vi "Get Error Source Components.vi"(11 "Error Source String":string) -> (1 "DQMH Error Hint":string, 2 "Call Chain":string[](array[string]), 3 "Error Message":string)   [LabVIEW 2024, in "hse-logger.lvlib" / "Formatter.lvclass"]
doc: "Extract the call chain from extended source strings.\n\n____\nHAMPEL SOFTWARE ENGINEERING v2.2.2 (2025-01-16 15:41)"
uses:
  <vilib>/Hampel Software Engineering/HSE Logger/Formatter/Formatter.lvclass
  <vilib>/Utility/error.llb/Trim Whitespace One-Sided.vi
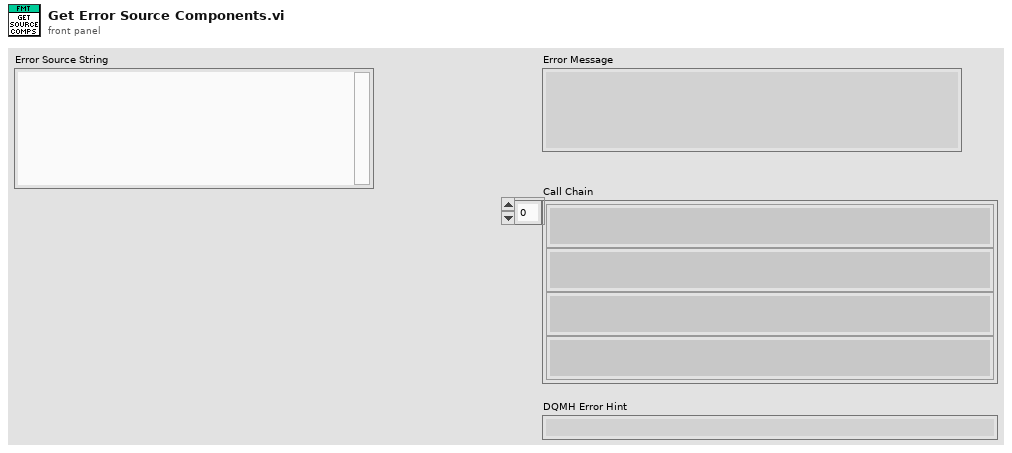
[diagram p1: front panel]
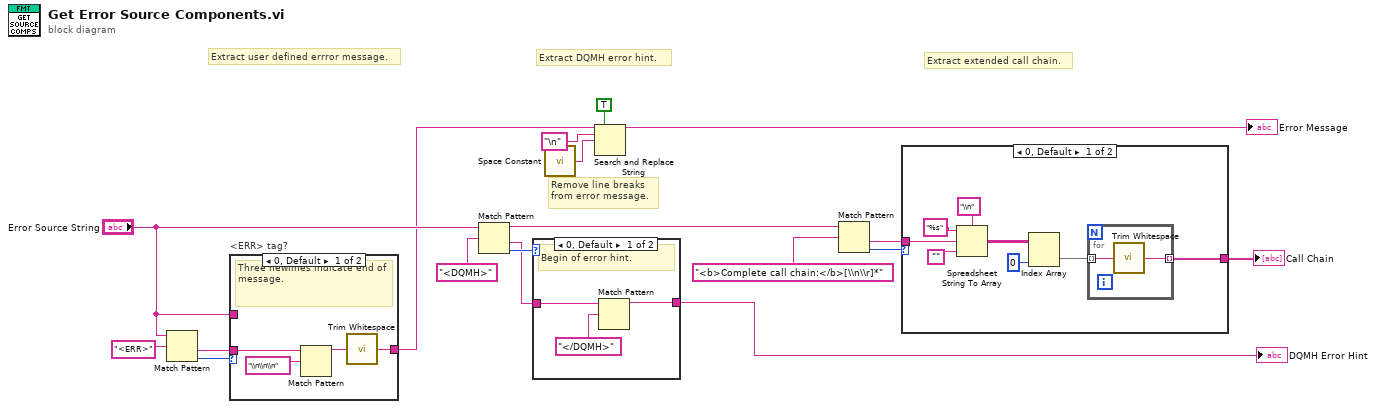
[diagram p0: block diagram]
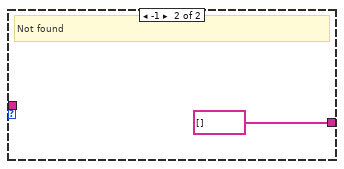
[diagram p4: hidden frame]
diagram:
  # "Remove line breaks\nfrom error message."
  # "Extract user defined errror message."
  # "Extract extended call chain."
  # "Extract DQMH error hint."
  n1 = Match Pattern(string="Error Source String", regular expression="<ERR>") -> (after substring=w9:string, offset past match=w8:i32)  [unwired: 1 in, 2 out]
  n2 = case "<ERR> tag?" shown="0, Default" w8 {
    tunnel: w9 -> [w22 _]
    tunnel: "Error Source String" -> [_ w23]
    tunnel: [w19 w23] -> w2
    frame 0, Default {
      # "Three newlines indicate end of message."
      n3 = Match Pattern(string=w22, regular expression="\\n\\n\\n") -> (before substring=w20:string)  [unwired: 1 in, 3 out]
      n4 = call <vilib>:"Trim Whitespace.vi"("string"=w20) -> ("trimmed string"=w19:string)  [unwired: 1 in]
    }
    frame -1 {
      # "No extended error information."
    }
  }
  n5 = Match Pattern(string="Error Source String", regular expression="<DQMH>") -> (before substring=w11:string, after substring=w12:string, offset past match=w13:i32)  [unwired: 1 in, 1 out]
  n6 = case shown="0, Default" w13 {
    tunnel: w12 -> [w26 w27]
    tunnel: [w24 w27] -> w10
    frame 0, Default {
      # "Begin of error hint."
      n7 = Match Pattern(string=w26, regular expression="</DQMH>") -> (before substring=w24:string)  [unwired: 1 in, 3 out]
    }
    frame -1 {
      # "Empty"
      # "No DQMH error hint."
    }
  }
  "DQMH Error Hint" <- w10
  n8 = call <vilib>:"Space Constant.vi"() -> ("String"=w1:string)
  n9 = Search and Replace String(replace all?=TRUE ("replace all? (F)"), input string=w2, search string="\n", replace string=w1) -> (result string=→"Error Message":string)  [unwired: 4 in, 3 out]
  n10 = Match Pattern(string=w11, regular expression="<b>Complete call chain:</b>[\\n\\r]*") -> (after substring=w16:string, offset past match=w17:i32)  [unwired: 1 in, 2 out]
  n11 = case shown="0, Default" w17 {
    tunnel: [w28 string[] []] -> w15
    tunnel: w16 -> [w35 _]
    frame 0, Default {
      n12 = Spreadsheet String To Array(delimiter (Tab)="\\n", format string="%s", spreadsheet string=w35, array type (2D Dbl)="") -> (array=w32:string[][])
      n13 = Index Array(array=w32, index (col)=0 ("disabled index (col)")) -> (element=w29:string[])  [unwired: 1 in]
      n14 = for {
        tunnel: w29 -> [w37] mode=indexing
        tunnel: [w36] -> w28 mode=indexing
        n15 = call <vilib>:"Trim Whitespace.vi"("string"=w37) -> ("trimmed string"=w36:string)  [unwired: 1 in]
      }
    }
    frame -1 {
      # "Not found"
    }
  }
  "Call Chain" <- w15
